vi "UART Open.vi"(8 "Error In":errorcluster, 9 "Baud Rate (9600)":u32=9600, 10 "UART Channel (0)":u8, 11 "LINX Resource":T1) -> (0 "Error Out":errorcluster, 2 "Actual Baud":u32, 3 "LINX Resource":T1)   [LabVIEW 2014, in "LMH-LINX.lvlib"]
doc: "Open the UART channel with the specified baud rate. If the LINX device has a single UART it is channel 0. If the LINX device has more than one UART the logical first UART is channel 0, the next is channel 1, etc.\n\nFor example on myRIO:\nA/UART maps to LINX UART Channel 0\nB/UART maps to LINX UART Channel 1"
uses:
  <vilib>/MakerHub/LINX/LMH-LINX.lvlib
  <vilib>/MakerHub/LINX/Private/Type Defs/LINX Ref.ctl
  <vilib>/MakerHub/LINX/Private/Type Defs/Platform.ctl
  <vilib>/MakerHub/LINX/Private/Type Defs/Interface.ctl
  <vilib>/MakerHub/LINX/Private/Device/Type Defs/LINX Device Config.ctl
  <vilib>/MakerHub/LINX/Private/Device/Type Defs/TCP Config.ctl
  <vilib>/MakerHub/LINX/Private/Device/Type Defs/Channels.ctl
  <vilib>/MakerHub/LINX/Private/Type Defs/Peripheral.ctl
  <vilib>/MakerHub/LINX/Private/Utilties/Generate Error.vi
  <vilib>/MakerHub/LINX/Private/Device/Device.lvlib
  <vilib>/MakerHub/LINX/Private/Local IO/Local IO.lvlib
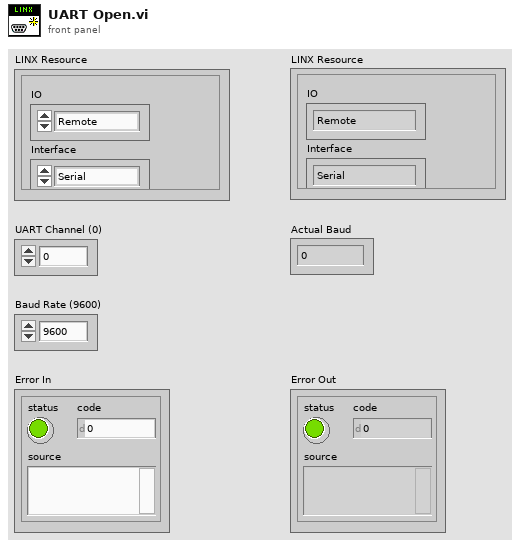
[diagram p1: front panel]
types:
  T1 = typedef "LMH-LINX.lvlib/LINX Ref.ctl" = cluster{"IO":T2, "Interface":T3, "LINX Device Config":T4}
  T2 = typedef "LMH-LINX.lvlib/Platform.ctl" = enum16{"Remote", "Local"}
  T3 = typedef "LMH-LINX.lvlib/Interface.ctl" = enum16{"Serial", "TCP"}
  T4 = typedef "LMH-LINX.lvlib/Device.lvlib/LINX Device Config.ctl" = cluster{"Interface":T3, "COM Port":refnum<visa-resource-name>, "TCP Configuration":T5, "Device Family":u8, "Device ID":u8, "Device Name":string, "TCP Ref":refnum<k5>, "Channels":T6}
  T5 = typedef "LMH-LINX.lvlib/Device.lvlib/TCP Config.ctl" = cluster{"IP Address":string, "Port":u16}
  T6 = typedef "LMH-LINX.lvlib/Channels.ctl" = cluster{"DI":u8[], "DO":u8[], "AI":u8[], "AO":u8[], "PWM":u8[], "QE":u8[], "UART":u8[], "I2C 2":u8[], "SPI":u8[], "CAN":u8[], "Servo":u8[], "AI Ref (V)":dbl, "AI Resolution (Bits)":u8, "AO Ref (V)":dbl, "AO Resolution (Bits)":u8}
  T7 = typedef "LMH-LINX.lvlib/Peripheral.ctl" = enum8{"DI", "DO", "AI", "AO", "PWM", "QE", "UART", "I2C", "SPI", "CAN", "Servo"}
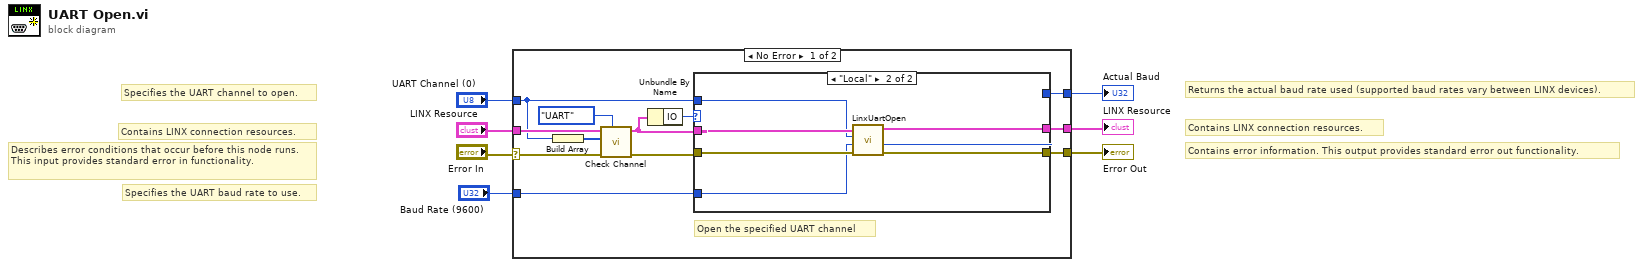
[diagram p0: block diagram]
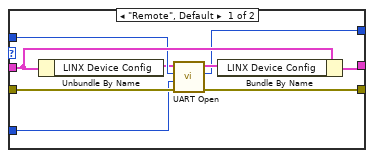
[diagram p2: hidden frame]
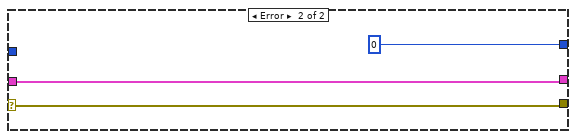
[diagram p3: hidden frame]
diagram:
  # "Returns the actual baud rate used (supported baud rates vary between LINX devices)."
  # "Specifies the UART baud rate to use."
  # "Specifies the UART channel to open."
  # "Contains LINX connection resources."
  # "Contains error information. This output provides standard error out functionality."
  # "Contains LINX connection resources."
  # "Describes error conditions that occur before this node runs. This input provides standard error in functionality."
  n1 = case shown="No Error" "Error In" {
    selector: "Error In" -> [w9 w38]
    tunnel: [w18 w38] -> w7
    tunnel: [w17 w37] -> w6
    tunnel: "LINX Resource" -> [w16 w37]
    tunnel: "UART Channel (0)" -> [w12 _]
    tunnel: "Baud Rate (9600)" -> [w10 _]
    tunnel: [w8 u32 0 ("Baud Rate (9600)")] -> w1
    frame No Error {
      # "Open the specified UART channel"
      n2 = Build Array(w12) -> (w13:u8[])
      n3 = call <vilib>:"Check Channel.vi"("Peripheral"=Peripheral."UART", "Error In"=w9, "Channels"=w13, "LINX Resource"=w16) -> ("Error Out"=w14:errorcluster, "LINX Resource"=w15:T1)  [unwired: 5 in, 1 out]
      n4 = Unbundle By Name(w15) -> ("IO"=w19:T2)
      n5 = case shown="\"Local\"" w19 {
        tunnel: w14 -> [w25 w35]
        tunnel: w15 -> [w28 w34]
        tunnel: [w26 w32] -> w18
        tunnel: [w27 w33] -> w17
        tunnel: w12 -> [w24 w30]
        tunnel: w10 -> [w23 w29]
        tunnel: [w20 w31] -> w8
        frame "Remote", Default {
          n6 = Unbundle By Name(w28) -> ("LINX Device Config"=w22:T4)
          n7 = call <vilib>:"UART Open.vi"("Error In"=w25, "Baud Rate (9600)"=w23, "UART Channel"=w24, "LINX Device Config"=w22) -> ("Error Out"=w26:errorcluster, "Actual Baud"=w20:u32, "LINX Device Config"=w21:T4)  [unwired: 5 in]
          n8 = Bundle By Name(cluster=w28, "LINX Device Config"=w21) -> (w27:T1)
        }
        frame "Local" {
          n9 = call <vilib>:"LinxUartOpen.vi"("Error In"=w35, "Baud Rate"=w29, "Uart Channel"=w30, "LINX Resource"=w34) -> ("Error Out"=w32:errorcluster, "Actual Baud Rate"=w31:u32, "LINX Resource"=w33:T1)  [unwired: 5 in]
        }
      }
    }
    frame Error {
    }
  }
  "Error Out" <- w7
  "LINX Resource" <- w6
  "Actual Baud" <- w1
